vi "Save States.vi"(8 "Error In":errorcluster, 9 "States Variant":variant, 10 "UIM Tag":refnum<k20>, 11 "XML Refnum":refnum<k20>) -> (0 "XML Error Out":errorcluster, 2 "UIM Tag Out":refnum<k20>, 3 "XML Refnum Out":refnum<k20>)   [LabVIEW 2020, in "UIM.lvlib" / "UIM.lvclass"]
uses:
  UIM.lvclass
  UIP Interface/UIP Interface.lvclass
  <vilib>/xml/Close Reference(Node).vi
  UIM.lvclass/UIM.ctl
  <vilib>/xml/NI_XML.lvlib
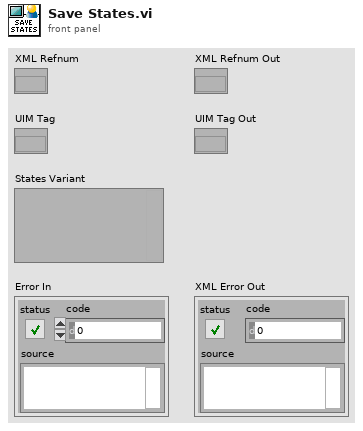
[diagram p1: front panel]
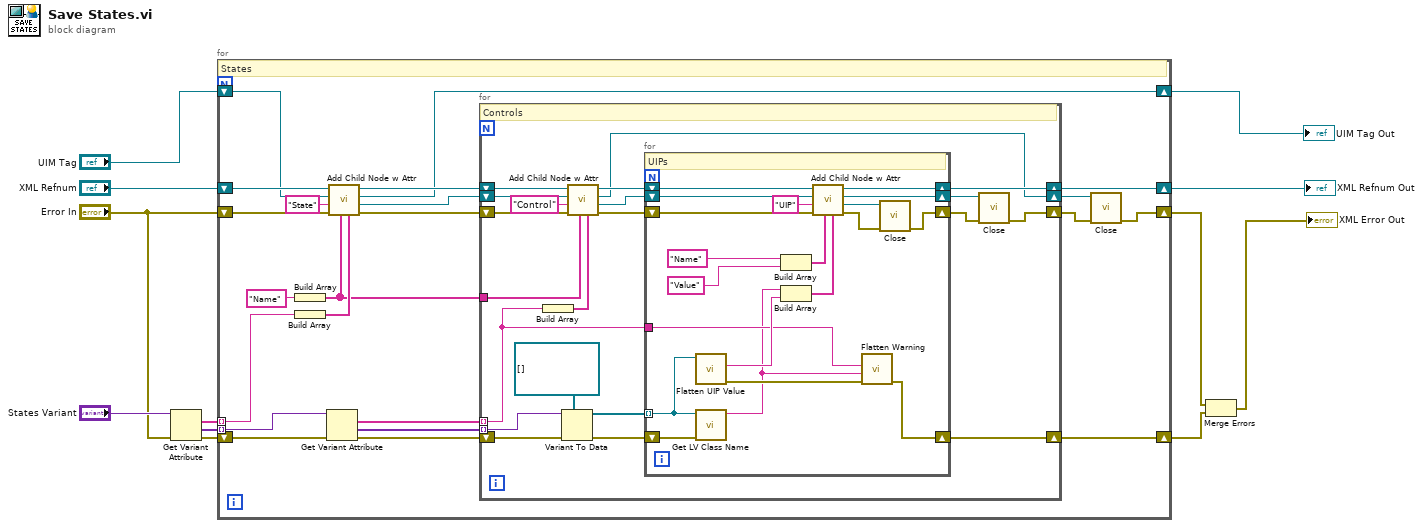
[diagram p0: block diagram]
diagram:
  n1 = Get Variant Attribute(Variant="States Variant", error in="Error In") -> (names=w12:string[], values=w11:variant[], error out=w10:errorcluster)  [unwired: 2 in, 1 out]
  n2 = for {
    tunnel: w12 -> [w32] mode=indexing
    tunnel: w11 -> [w16] mode=indexing
    shift-right: [w23] -> w7
    shift-left: w10 -> [w17]
    shift-right: [w18] -> w1
    shift-left: "Error In" -> [w29]
    shift-right: [w24] -> w8
    shift-left: "XML Refnum" -> [w34]
    shift-right: [w19] -> w2
    shift-left: "UIM Tag" -> [w31]
    # "States"
    n3 = Build Array("Name" ("Name")) -> (w25:string[])
    n4 = Build Array(w32) -> (w28:string[])
    n5 = Get Variant Attribute(Variant=w16, error in=w17) -> (names=w15:string[], values=w14:variant[], error out=w13:errorcluster)  [unwired: 2 in, 1 out]
    n6 = call "Add Child Node w Attr.vi"("Values"=w28, "Names"=w25, "Error In"=w29, "Tag Name"="State", "Parent Node"=w31, "DOM In"=w34) -> ("Error Out"=w26:errorcluster, "Child Node"=w22:refnum<k20>, "Parent Node"=w19:refnum<k20>, "DOM Out"=w27:refnum<k20>)  [unwired: 2 in]
    n7 = for {
      tunnel: w14 -> [w54] mode=indexing
      tunnel: w15 -> [w35] mode=indexing
      shift-right: [w42] -> w23
      shift-left: w13 -> [w53]
      tunnel: w25 -> [w47]
      shift-right: [w37] -> w20
      shift-left: w26 -> [w49]
      shift-right: [w43] -> w24
      shift-left: w27 -> [w51]
      shift-right: [w38] -> w21
      shift-left: w22 -> [w50]
      # "Controls"
      n8 = Build Array(w35) -> (w46:string[])
      n9 = Variant To Data(error in=w53, type=refnum<class "UIP Interface.lvclass">[] [] ("UIP Defs"), Variant=w54) -> (data=w52:refnum<class "UIP Interface.lvclass">[], error out=w36:errorcluster)
      n10 = call "Add Child Node w Attr.vi"("Values"=w46, "Names"=w47, "Error In"=w49, "Tag Name"="Control", "Parent Node"=w50, "DOM In"=w51) -> ("Error Out"=w44:errorcluster, "Child Node"=w41:refnum<k20>, "Parent Node"=w38:refnum<k20>, "DOM Out"=w45:refnum<k20>)  [unwired: 2 in]
      n11 = for {
        tunnel: w52 -> [w75] mode=indexing
        shift-right: [w65] -> w40
        shift-left: w44 -> [w73]
        shift-right: [w64] -> w43
        shift-left: w45 -> [w74]
        shift-right: [w57] -> w42
        shift-left: w36 -> [w60]
        shift-right: [w62] -> w39
        shift-left: w41 -> [w63]
        tunnel: w35 -> [w58]
        # "UIPs"
        n12 = call-dynamic "Flatten UIP Value.vi"("UIP In"=w75) -> ("Error Out"=w59:errorcluster, "String Value"=w68:string)  [unwired: 8 in, 1 out]
        n13 = call <vilib>:"Get LV Class Name.vi"("error in (no error)"=w60, "object"=w75) -> ("class name"=w56:string)  [unwired: 8 in, 1 out]
        n14 = Build Array("Name" ("Name"), "Value" ("Name")) -> (w69:string[])
        n15 = Build Array(w56, w68) -> (w67:string[])
        n16 = call "Add Child Node w Attr.vi"("Values"=w67, "Names"=w69, "Error In"=w73, "Tag Name"="UIP", "Parent Node"=w63, "DOM In"=w74) -> ("Error Out"=w66:errorcluster, "Child Node"=w61:refnum<k20>, "Parent Node"=w62:refnum<k20>, "DOM Out"=w64:refnum<k20>)  [unwired: 2 in]
        n17 = call "Flatten Warning.vi"("Error In"=w59, "UIP Name"=w56, "Label.Text"=w58) -> ("Error Out"=w57:errorcluster)  [unwired: 8 in]
        n18 = call-poly <vilib>:"Close.vi"("error in (no error)"=w66, "node"=w61) -> ("error out"=w65:errorcluster)  [unwired: 7 in]
      }
      n19 = call-poly <vilib>:"Close.vi"("error in (no error)"=w40, "node"=w39) -> ("error out"=w37:errorcluster)  [unwired: 7 in]
    }
    n20 = call-poly <vilib>:"Close.vi"("error in (no error)"=w20, "node"=w21) -> ("error out"=w18:errorcluster)  [unwired: 7 in]
  }
  "XML Refnum Out" <- w8
  "UIM Tag Out" <- w2
  n21 = Merge Errors(w1, w7) -> (→"XML Error Out":errorcluster)
